vi "logbookEntry.vi"(0 "Log book entry":string) -> (1 "Log book path":string, 2 "folderPresent":bool)   [LabVIEW 2017]
uses:
  globalUtilities.vi
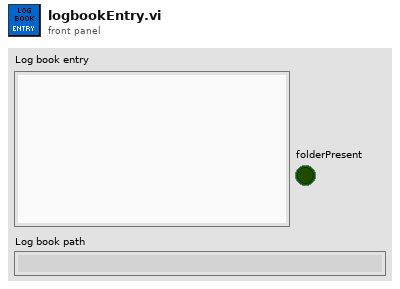
[diagram p1: front panel]
types:
  T1 = enum16{"open", "replace", "create", "open or create", "replace or create", "replace or create with confirmation"}
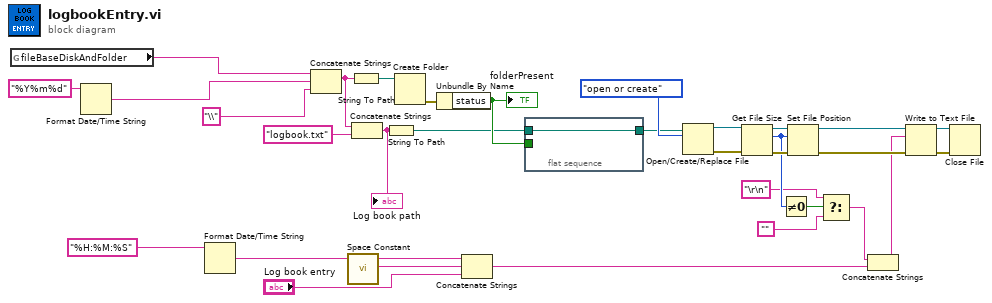
[diagram p0: block diagram]
diagram:
  n1 = global read "globalUtilities.vi" "fileBaseDiskAndFolder"() -> (w17:string)
  n2 = Format Date/Time String(time format string (%c)="%Y%m%d") -> (date/time string=w16:string)  [unwired: 2 in]
  n3 = Format Date/Time String(time format string (%c)="%H:%M:%S") -> (date/time string=w12:string)  [unwired: 2 in]
  n4 = Concatenate Strings(w17, w16, "\\") -> (w15:string)
  n5 = call <vilib>:"Space Constant.vi"() -> ("String"=w11:string)
  n6 = String To Path(string=w15) -> (path=w13:path)
  n7 = Concatenate Strings(w15, "logbook.txt" ("string")) -> (w14:string)
  "Log book path" <- w14
  n8 = String To Path(string=w14) -> (path=w2:path)
  n9 = Create Folder(path (use dialog)=w13) -> (error out=w5:errorcluster)  [unwired: 2 in, 2 out]
  n10 = Unbundle By Name(w5) -> ("status"=w3:bool)
  "folderPresent" <- w3
  n11 = Concatenate Strings(w12, w11, "Log book entry") -> (w4:string)
  n12 = flat-sequence {
    tunnel: w3 -> [_]
    tunnel: w2 -> [w33]
    tunnel: [w33] -> w1
    frame #0 {
    }
  }
  n13 = Open/Create/Replace File(file path (use dialog)=w1, operation (0:open)=T1."open or create") -> (refnum out=w32:refnum<file>, error out=w31:errorcluster)  [unwired: 4 in, 1 out]
  n14 = Get File Size(file=w32, error in=w31) -> (refnum out=w29:refnum<file>, size (in bytes)=w23:i64, 0:w30:errorcluster)
  n15 = Not Equal To 0?(x=w23) -> (x != 0?=w22:bool)
  n16 = Set File Position(offset (in bytes) (0)=w23, refnum=w29, error in=w30) -> (refnum out=w28:refnum<file>, error out=w27:errorcluster)  [unwired: 1 in]
  n17 = Select(t="\r\n", s=w22, f="") -> (s? t:f=w19:string)
  n18 = Concatenate Strings(w19, w4) -> (w18:string)
  n19 = Write to Text File(file (use dialog)=w28, text=w18, error in=w27) -> (refnum out=w26:refnum<file>, error out=w25:errorcluster)  [unwired: 1 in, 1 out]
  n20 = Close File(refnum=w26, error in=w25) -> ()  [unwired: 2 out]
